vi "Get One VR Crank Revolution Data.vi"(11 "Data In":dbl[](array[numeric])) -> (3 "One VR Crank Period":dbl[](array[numeric]), 5 "Selected Length":i32, 7 "Selected Offset":i32)   [LabVIEW 2011, in "Engine Sim System Explorer.lvlib"]
uses:
  Engine Sim System Explorer.lvlib
  <vilib>/ptbypt/NI_PtbyPt.lvlib
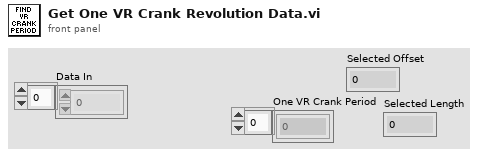
[diagram p1: front panel]
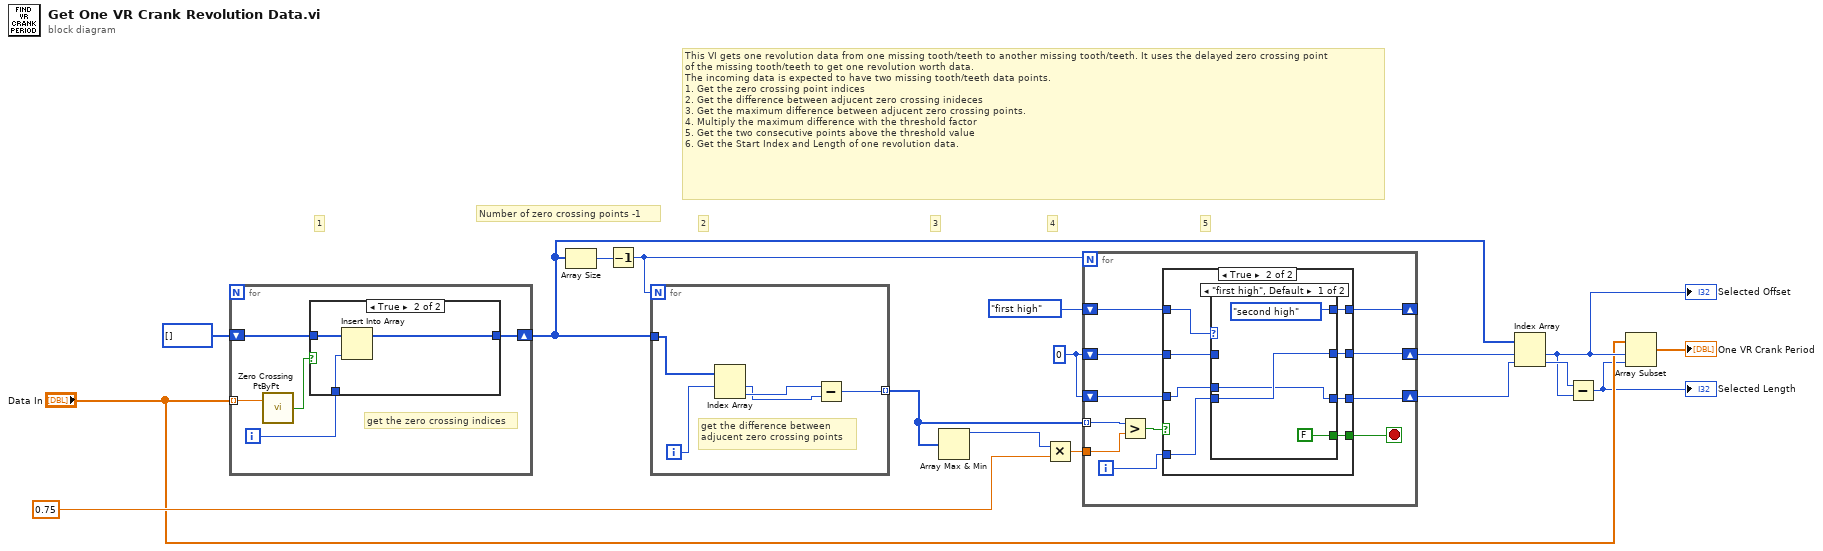
[diagram p0: block diagram]
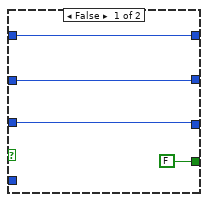
[diagram p2: hidden frame]
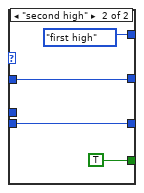
[diagram p3: hidden frame]
diagram:
  w17 = 0
  # "5"
  # "Number of zero crossing points -1"
  # "4"
  # "3"
  # "2"
  # "1"
  # "This VI gets one revolution data from one missing tooth/teeth to another missing tooth/teeth. It uses the delayed zero crossing point\nof the missing tooth/teeth to get one revolution worth data. \nThe incoming data is expected to have two missing tooth/teeth data points.\n1. Get the zero crossing point indices\n2. Get the difference between adjucent zero crossing inideces\n3. Get the maximum difference between adjucent zero crossing points.\n4. Multiply the maximum difference with the threshold factor\n5. Get the two consecutive points above the threshold value\n6. Get the Start Index and Length of one revolution data."
  n1 = for {
    tunnel: "Data In" -> [w22] mode=indexing
    shift-right: [w18] -> w7
    shift-left: i32[] [] -> [w20]
    i -> [w19]
    # "get the zero crossing indices"
    n2 = call <vilib>:"Zero Crossing PtByPt.vi"("input data point"=w22) -> ("crossing"=w21:bool)  [unwired: 2 in]
    n3 = case shown="True" w21 {
      tunnel: w20 -> [w23 w26]
      tunnel: w19 -> [_ w25]
      tunnel: [w23 w24] -> w18
      frame False {
      }
      frame True {
        n4 = Insert Into Array(array=w26, new element=w25) -> (w24:i32[])  [unwired: 1 in]
      }
    }
  }
  n5 = Array Size(array=w7) -> (size(s)=w12:i32)
  n6 = Decrement(x=w12) -> (x-1=w5:i32)
  n7 = for {
    N: w5 -> [_]
    tunnel: w7 -> [w27]
    tunnel: [w28] -> w6 mode=indexing
    i -> [w31]
    # "get the difference between\nadjucent zero crossing points"
    n8 = Index Array(array=w27, index #1=w31) -> (element #1=w29:i32, element #2=w30:i32)  [unwired: 1 in]
    n9 = Subtract(x=w30, y=w29) -> (x-y=w28:i32)
  }
  n10 = Array Max & Min(array=w6) -> (max value=w13:i32)  [unwired: 3 out]
  n11 = Multiply(x=w13, y=sgl 0.75 ("Threshold Factor")) -> (x*y=w15:sgl)
  n12 = for {
    N: w5 -> [_]
    tunnel: w6 -> [w42] mode=indexing
    tunnel: w15 -> [w41]
    shift-right: [w36] -> _
    shift-left: enum16{"first high", "second high"}."first high" -> [w39]
    shift-right: [w37] -> w10
    shift-left: w17 -> [w34]
    shift-right: [w35] -> w9
    shift-left: w17 -> [w33]
    i -> [w38]
    stop <- w32 stop-if-true
    n13 = Greater?(x=w42, y=w41) -> (0:w40:bool)
    n14 = case shown="True" w40 {
      tunnel: w39 -> [w46 w54]
      tunnel: w38 -> [_ w53]
      tunnel: [w45 w52] -> w37
      tunnel: [w46 w51] -> w36
      tunnel: [w44 w50] -> w35
      tunnel: w34 -> [w45 w49]
      tunnel: w33 -> [w44 w48]
      tunnel: [FALSE w47] -> w32
      frame False {
      }
      frame True {
        n15 = case shown="\"first high\", Default" w54 {
          tunnel: w53 -> [w58 w62]
          tunnel: [w58 w61] -> w52
          tunnel: [enum16{"first high", "second high"}."second high" enum16{"first high", "second high"}."first high"] -> w51
          tunnel: [w56 w62] -> w50
          tunnel: w49 -> [_ w61]
          tunnel: w48 -> [w56 _]
          tunnel: [FALSE TRUE] -> w47
          frame "first high", Default {
          }
          frame "second high" {
          }
        }
      }
    }
  }
  n16 = Index Array(array=w7, index #1=w10, index #2=w9) -> (element #1=w4:i32, element #2=w8:i32)
  "Selected Offset" <- w4
  n17 = Subtract(x=w8, y=w4) -> (x-y=w1:i32)
  "Selected Length" <- w1
  n18 = Array Subset(array="Data In", index=w4, length=w1) -> (→"One VR Crank Period":dbl[])
